vi "VisionGetCamerasConnected.vi"() -> (1 "Vision Connected Right":bool, 3 "Vision Connected Left":bool)   [LabVIEW 2023]
doc: "gets current position"
uses:
  VisionGlobal.vi
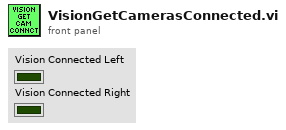
[diagram p1: front panel]
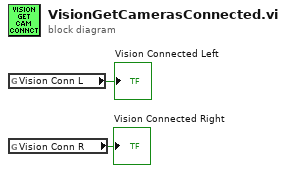
[diagram p0: block diagram]
diagram:
  n1 = global read "VisionGlobal.vi" "Vision Conn L"() -> (→"Vision Connected Left":bool)
  n2 = global read "VisionGlobal.vi" "Vision Conn R"() -> (→"Vision Connected Right":bool)
